vi "frontp_generate_hardware_seqs.vi"(8 "error in (no error)":errorcluster, 11 "front_panel in":refnum<class "front_panel.lvclass">) -> (0 "error out":errorcluster, 3 "front_panel out":refnum<class "front_panel.lvclass">)   [LabVIEW 2015, in "front_panel.lvclass"]
uses:
  front_panel.lvclass
  Hardware Class/hardware/hardware.lvclass
  panel_class/panel.lvclass
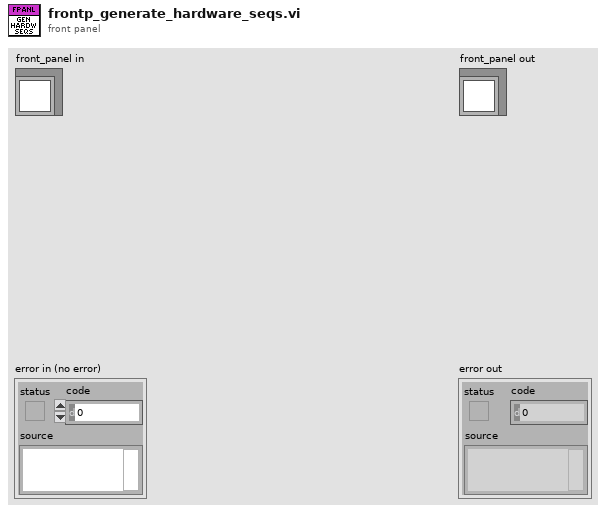
[diagram p1: front panel]
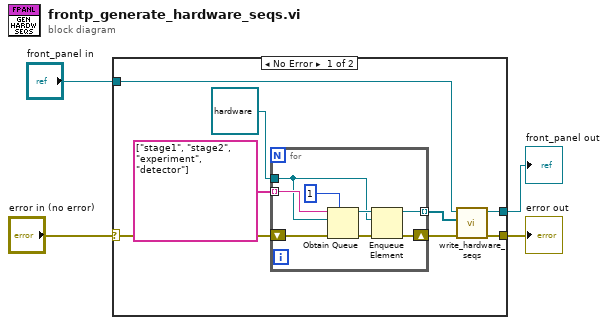
[diagram p0: block diagram]
diagram:
  n1 = case shown="No Error" "error in (no error)" {
    selector: "error in (no error)" -> [w11 w22]
    tunnel: [w8 w22] -> w3
    tunnel: [w7 w21] -> w1
    tunnel: "front_panel in" -> [w6 w21]
    frame No Error {
      n2 = for {
        tunnel: string[] ["stage1", "stage2", "experiment", "detector"] -> [w18] mode=indexing
        shift-right: [w16] -> w9
        shift-left: w11 -> [w17]
        tunnel: [w15] -> w5 mode=indexing
        tunnel: refnum<class "hardware.lvclass"> refnum ("hardware.lvclass") -> [w14]
        n3 = Obtain Queue(max queue size (-1, unlimited)=1, name (unnamed)=w18, element data type=w14, error in (no error)=w17) -> (queue out=w19:refnum<queue>, error out=w20:errorcluster)  [unwired: 1 in, 1 out]
        n4 = Enqueue Element(queue=w19, element=w14, error in (no error)=w20) -> (queue out=w15:refnum<queue>, error out=w16:errorcluster)  [unwired: 1 in, 1 out]
      }
      n5 = call "write_hardware_seqs.vi"("error in (no error)"=w9, "hardware_SEQs"=w5, "panel in"=w6) -> ("error out"=w8:errorcluster, "panel out"=w7:refnum<class "front_panel.lvclass">)  [unwired: 7 in]
    }
    frame Error {
    }
  }
  "error out" <- w3
  "front_panel out" <- w1
